vi "Load and Vin SMU Measurement.vi"() -> ()   [LabVIEW 2021]
doc: "Demonstrates how to use the DC Voltage Output Function to force an output voltage. This example initializes a session, configures the Output Function, Sense, Autorange, Voltage Level and Current Limit, initiates generation, waits for a specified delay, and measures the voltage and current output. This example uses Single Point source mode."
uses:
  <instrlib>/niDMM/nidmm.llb/niDMM Function.ctl
  <instrlib>/niDMM/nidmm.llb/niDMM Resolution in Digits.ctl
  <instrlib>/niDCPower/nidcpower.llb/niDCPower Output Function.ctl
  <instrlib>/niDCPower/nidcpower.llb/niDCPower Source Mode.ctl
  <instrlib>/niDMM/nidmm.llb/niDMM Configure Measurement Digits.vi
  <instrlib>/Tektronix MSO5X Series/Tektronix MSO5X Series.lvlib
panel:
  in  "Tektronix Scope":refnum<visa-resource-name>
  out "Division Number":i32
  in  "Sample Rate":dbl=3125000000.0
  in  "Maximum Record Length":dbl=250000000.0 format="%#_6e"
  out "SMU Measurement":dbl format="%.6p"
  in  "SMU DMM":refnum<k15>="Dev1"
  in  "SMU DMM Measurement":T1
  in  "SMU Resolution in Digits":T2=5.5 items=["3 1/2"=3.5, "4 1/2"=4.5, "5 1/2"=5.5, "6 1/2"=6.5, "7 1/2"=7.5]
  out "Load Voltage":dbl caption="SMU Measurement" format="%.6p"
  in  "Load DMM":refnum<k15>="Dev1"
  in  "Load DMM Measurement":T1 caption="SMU DMM Measurement"
  in  "Load SMU":refnum<k15>="Dev1"
  in  "Load SMU Channel":string="0"
  out "Load SMU Current":dbl
  out "Load SMU Voltage":dbl
  in  "error in":errorcluster
  out "error out":errorcluster
  out "Voltage Measurement":dbl caption="Vin SMU Voltage"
  out "Current Measurement":dbl caption="Vin SMU Current"
  in  "Current Limit":dbl=0.01 format="%.3p"
  in  "Voltage Level":dbl=2.0 format="%.5p"
  in  "Vin SMU Channel":string="0"
  in  "Vin SMU":refnum<k15>="Dev1"
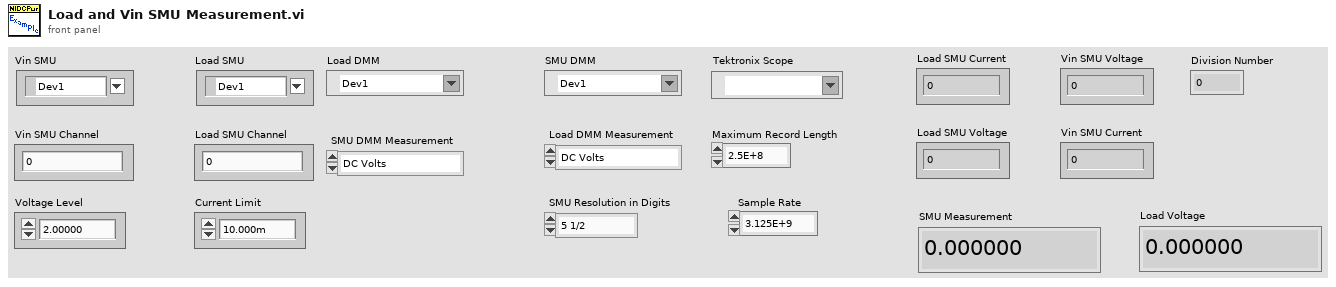
[diagram p1: front panel]
types:
  T1 = typedef "niDMM Function.ctl" = enum16{"DC Volts", "AC Volts", "DC Current", "AC Current", "2-wire Resistance", "4-wire Resistance", "Diode", "Frequency", "Period", "AC Volts DC Coupled", "Capacitance", "Inductance", "Temperature"}
  T2 = typedef "niDMM Resolution in Digits.ctl" = dbl
  T3 = typedef "niDCPower Output Function.ctl" = i32
  T4 = typedef "niDCPower Source Mode.ctl" = i32
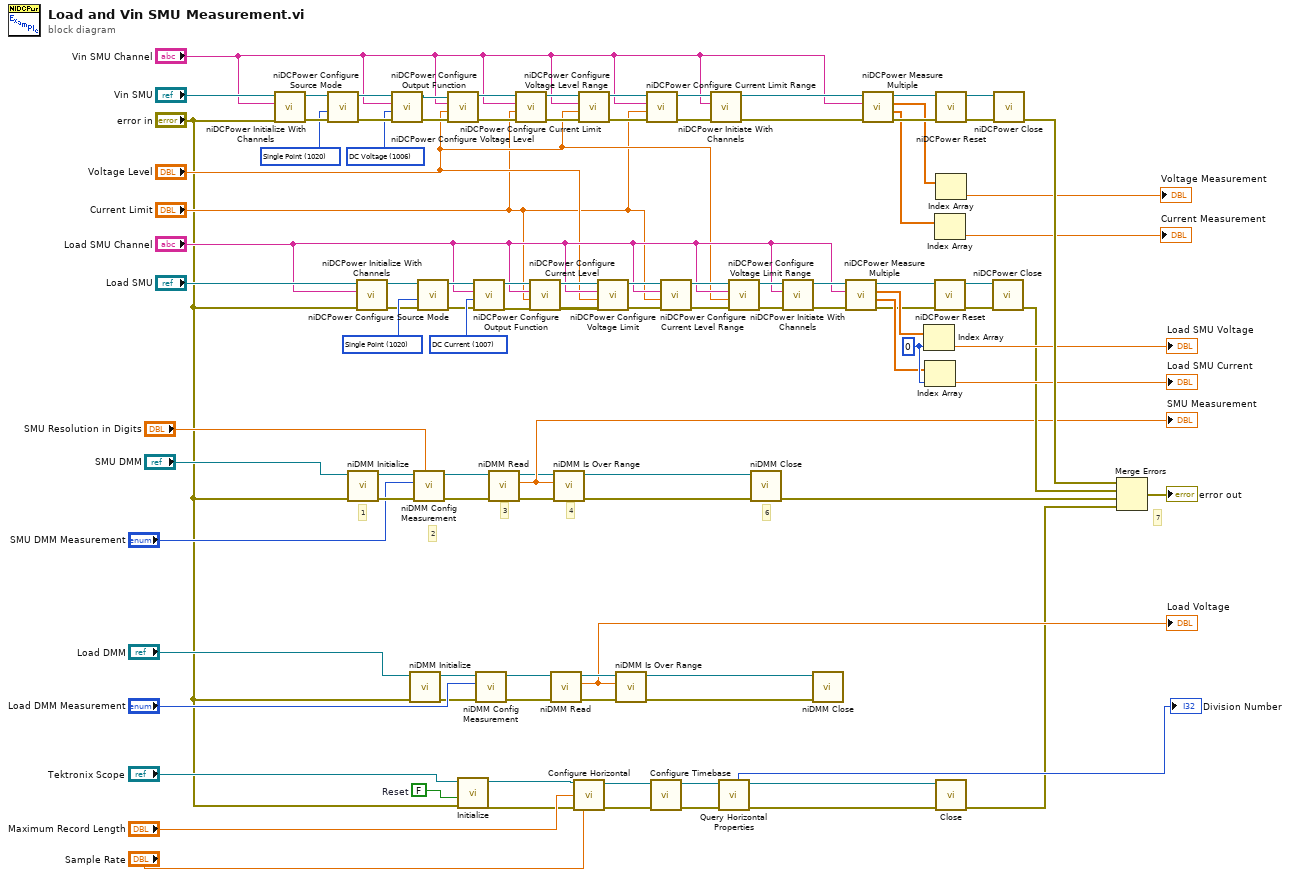
[diagram p0: block diagram]
diagram:
  w6 = FALSE  # Reset
  w73 = T3 1007 items=["DC Voltage"=1006, "DC Current"=1007, "Pulse Voltage"=1049, "Pulse Current"=1050] ("output function")
  w64 = 0 ("index")
  w55 = T4 1020 items=["Single Point"=1020, "Sequence"=1021] ("source mode")
  w79 = T3 1006 items=["DC Voltage"=1006, "DC Current"=1007, "Pulse Voltage"=1049, "Pulse Current"=1050] ("output function")
  w92 = T4 1020 items=["Single Point"=1020, "Sequence"=1021] ("source mode")
  # "2"
  # "1"
  # "7"
  # "6"
  # "4"
  # "3"
  n1 = call <instrlib>:"niDCPower Initialize With Channels.vi"("error in (no error)"="error in", "channels"="Vin SMU Channel", "resource name"="Vin SMU") -> ("error out"=w96:errorcluster, "instrument handle out"=w95:refnum<k15>)  [unwired: 2 in, 5 out]
  n2 = call <instrlib>:"niDCPower Configure Source Mode.vi"("error in (no error)"=w96, "source mode"=w92, "instrument handle"=w95) -> ("error out"=w94:errorcluster, "instrument handle out"=w93:refnum<k15>)  [unwired: 7 out]
  n3 = call <instrlib>:"niDMM Initialize.vi"("error in (no error)"="error in", "Instrument Descriptor"="SMU DMM") -> ("error out"=w26:errorcluster, "instrument handle out"=w27:refnum<k15>)  [unwired: 8 in]
  n4 = call <instrlib>:"niDCPower Initialize With Channels.vi"("error in (no error)"="error in", "channels"="Load SMU Channel", "resource name"="Load SMU") -> ("error out"=w51:errorcluster, "instrument handle out"=w52:refnum<k15>)  [unwired: 2 in, 5 out]
  n5 = call <instrlib>:"niDCPower Configure Output Function.vi"("error in (no error)"=w94, "output function"=w79, "channel name"="Vin SMU Channel", "instrument handle"=w93) -> ("error out"=w80:errorcluster, "instrument handle out"=w81:refnum<k15>)  [unwired: 6 out]
  n6 = call <instrlib>:"niDMM Initialize.vi"("error in (no error)"="error in", "Instrument Descriptor"="Load DMM") -> ("error out"=w32:errorcluster, "instrument handle out"=w31:refnum<k15>)  [unwired: 8 in]
  n7 = call-poly <instrlib>:"niDMM Config Measurement.vi"("Resolution in Digits"="SMU Resolution in Digits", "error in (no error)"=w26, "Function"="SMU DMM Measurement", "instrument handle"=w27) -> ("error out"=w20:errorcluster, "instrument handle out"=w21:refnum<k15>)  [unwired: 6 in]
  n8 = call <instrlib>:"niDCPower Configure Source Mode.vi"("error in (no error)"=w51, "source mode"=w55, "instrument handle"=w52) -> ("error out"=w53:errorcluster, "instrument handle out"=w54:refnum<k15>)  [unwired: 7 out]
  n9 = call <instrlib>:"niDCPower Configure Voltage Level.vi"("error in (no error)"=w80, "voltage level"="Voltage Level", "channel name"="Vin SMU Channel", "instrument handle"=w81) -> ("error out"=w99:errorcluster, "instrument handle out"=w100:refnum<k15>)  [unwired: 6 out]
  n10 = call <instrlib>:"Initialize.vi"("error in (no error)"="error in", "Reset (True)"=w6, "VISA resource name"="Tektronix Scope") -> ("error out"=w8:errorcluster, "VISA resource name out"=w7:refnum<visa-resource-name>)  [unwired: 7 in]
  n11 = call <instrlib>:"niDCPower Configure Output Function.vi"("error in (no error)"=w53, "output function"=w73, "channel name"="Load SMU Channel", "instrument handle"=w54) -> ("error out"=w71:errorcluster, "instrument handle out"=w72:refnum<k15>)  [unwired: 6 out]
  n12 = call-poly <instrlib>:"niDMM Config Measurement.vi"("error in (no error)"=w32, "Function"="Load DMM Measurement", "instrument handle"=w31) -> ("error out"=w38:errorcluster, "instrument handle out"=w37:refnum<k15>)  [unwired: 7 in]
  n13 = call <instrlib>:"niDMM Read.vi"("error in (no error)"=w20, "instrument handle"=w21) -> ("error out"=w23:errorcluster, "Measurement"=w24:dbl, "instrument handle out"=w22:refnum<k15>)  [unwired: 7 in]
  "SMU Measurement" <- w24
  n14 = call <instrlib>:"niDCPower Configure Current Limit.vi"("error in (no error)"=w99, "current limit"="Current Limit", "channel name"="Vin SMU Channel", "instrument handle"=w100) -> ("error out"=w91:errorcluster, "instrument handle out"=w90:refnum<k15>)  [unwired: 1 in, 5 out]
  n15 = call <instrlib>:"niDCPower Configure Current Level.vi"("error in (no error)"=w71, "current level"="Current Limit", "channel name"="Load SMU Channel", "instrument handle"=w72) -> ("error out"=w48:errorcluster, "instrument handle out"=w47:refnum<k15>)  [unwired: 6 out]
  n16 = call <instrlib>:"niDMM Read.vi"("error in (no error)"=w38, "instrument handle"=w37) -> ("error out"=w35:errorcluster, "Measurement"=w34:dbl, "instrument handle out"=w36:refnum<k15>)  [unwired: 7 in]
  "Load Voltage" <- w34
  n17 = call <instrlib>:"niDMM Is Over Range.vi"("error in (no error)"=w23, "Measurement"=w24, "instrument handle"=w22) -> ("error out"=w1:errorcluster, "instrument handle out"=w28:refnum<k15>)  [unwired: 6 in, 1 out]
  n18 = call <instrlib>:"Configure Horizontal.vi"("VISA resource name"=w7, "Maximum Record Length (2.5E+8)"="Maximum Record Length", "error in (no error)"=w8, "Sample Rate (3.125E+9)"="Sample Rate") -> ("VISA resource name out"=w14:refnum<visa-resource-name>, "error out"=w15:errorcluster)  [unwired: 10 in]
  n19 = call <instrlib>:"niDCPower Configure Voltage Level Range.vi"("error in (no error)"=w91, "voltage level range"="Voltage Level", "channel name"="Vin SMU Channel", "instrument handle"=w90) -> ("error out"=w89:errorcluster, "instrument handle out"=w88:refnum<k15>)  [unwired: 6 out]
  n20 = call <instrlib>:"niDCPower Configure Voltage Limit.vi"("error in (no error)"=w48, "voltage limit"="Voltage Level", "channel name"="Load SMU Channel", "instrument handle"=w47) -> ("error out"=w56:errorcluster, "instrument handle out"=w57:refnum<k15>)  [unwired: 6 out]
  n21 = call <instrlib>:"niDMM Is Over Range.vi"("error in (no error)"=w35, "Measurement"=w34, "instrument handle"=w36) -> ("error out"=w2:errorcluster, "instrument handle out"=w30:refnum<k15>)  [unwired: 6 in, 1 out]
  n22 = call <instrlib>:"niDCPower Configure Current Limit Range.vi"("error in (no error)"=w89, "current limit range"="Current Limit", "channel name"="Vin SMU Channel", "instrument handle"=w88) -> ("error out"=w84:errorcluster, "instrument handle out"=w85:refnum<k15>)  [unwired: 6 out]
  n23 = call <instrlib>:"Configure Timebase.vi"("error in (no error)"=w15, "VISA resource name"=w14) -> ("error out"=w16:errorcluster, "VISA resource name out"=w17:refnum<visa-resource-name>)  [unwired: 8 in]
  n24 = call <instrlib>:"niDCPower Configure Current Level Range.vi"("error in (no error)"=w56, "current level range"="Current Limit", "channel name"="Load SMU Channel", "instrument handle"=w57) -> ("error out"=w58:errorcluster, "instrument handle out"=w59:refnum<k15>)  [unwired: 6 out]
  n25 = call <instrlib>:"niDCPower Initiate With Channels.vi"("error in (no error)"=w84, "channel name"="Vin SMU Channel", "instrument handle"=w85) -> ("error out"=w82:errorcluster, "instrument handle out"=w83:refnum<k15>)  [unwired: 7 in]
  n26 = call <instrlib>:"Query Horizontal Properties.vi"("error in (no error)"=w16, "VISA resource name"=w17) -> ("error out"=w13:errorcluster, "VISA resource name out"=w12:refnum<visa-resource-name>, "Division Number"=→"Division Number":i32)  [unwired: 5 in, 2 out]
  n27 = call <instrlib>:"niDCPower Configure Voltage Limit Range.vi"("error in (no error)"=w58, "voltage limit range"="Voltage Level", "channel name"="Load SMU Channel", "instrument handle"=w59) -> ("error out"=w68:errorcluster, "instrument handle out"=w67:refnum<k15>)  [unwired: 6 out]
  n28 = call <instrlib>:"niDMM Close.vi"("error in (no error)"=w1, "instrument handle"=w28) -> ("error out"=w18:errorcluster)  [unwired: 9 in]
  n29 = call <instrlib>:"niDCPower Initiate With Channels.vi"("error in (no error)"=w68, "channel name"="Load SMU Channel", "instrument handle"=w67) -> ("error out"=w70:errorcluster, "instrument handle out"=w69:refnum<k15>)  [unwired: 7 in]
  n30 = call <instrlib>:"niDMM Close.vi"("error in (no error)"=w2, "instrument handle"=w30) -> ()  [unwired: 9 in, 1 out]
  n31 = call <instrlib>:"niDCPower Measure Multiple.vi"("error in (no error)"=w70, "channel name"="Load SMU Channel", "instrument handle"=w69) -> ("error out"=w61:errorcluster, "current measurements"=w63:dbl[], "voltage measurements"=w62:dbl[], "instrument handle out"=w60:refnum<k15>)  [unwired: 5 out]
  n32 = call <instrlib>:"niDCPower Measure Multiple.vi"("error in (no error)"=w82, "channel name"="Vin SMU Channel", "instrument handle"=w83) -> ("error out"=w86:errorcluster, "current measurements"=w77:dbl[], "voltage measurements"=w75:dbl[], "instrument handle out"=w87:refnum<k15>)  [unwired: 5 out]
  n33 = Index Array(array=w62, index=w64) -> (element=→"Load SMU Voltage":dbl)
  n34 = Index Array(array=w63, index=w64) -> (element=→"Load SMU Current":dbl)
  n35 = Index Array(array=w77) -> (element=→"Current Measurement":dbl)  [unwired: 1 in]
  n36 = call <instrlib>:"niDCPower Reset.vi"("error in (no error)"=w61, "instrument handle"=w60) -> ("error out"=w50:errorcluster, "instrument handle out"=w49:refnum<k15>)  [unwired: 2 in, 6 out]
  n37 = call <instrlib>:"niDCPower Reset.vi"("error in (no error)"=w86, "instrument handle"=w87) -> ("error out"=w97:errorcluster, "instrument handle out"=w98:refnum<k15>)  [unwired: 2 in, 6 out]
  n38 = Index Array(array=w75) -> (element=→"Voltage Measurement":dbl)  [unwired: 1 in]
  n39 = call <instrlib>:"Close.vi"("error in (no error)"=w13, "VISA resource name"=w12) -> ("error out"=w3:errorcluster)  [unwired: 9 in]
  n40 = call <instrlib>:"niDCPower Close.vi"("error in (no error)"=w50, "instrument handle"=w49) -> ("error out"=w44:errorcluster)  [unwired: 9 out]
  n41 = call <instrlib>:"niDCPower Close.vi"("error in (no error)"=w97, "instrument handle"=w98) -> ("error out"=w78:errorcluster)  [unwired: 9 out]
  n42 = Merge Errors(w78, w44, w18, w3) -> (→"error out":errorcluster)
